vi "CRYAdd curve name.vi"(9 "Curent Name":u16(ring) caption="aa" items=["Recalled Curve1"], 10 "add/rename?":bool, 11 "Curve Names in":string[](array[string])) -> (3 "Curve Names out":string[](array[string]))   [LabVIEW 2013]
panel:
  out "dialog text":string
  in  "Cancel":bool
  in  "OK":bool
  in  "New":bool caption="aa"
  in  "Custom Name":string caption="aa"
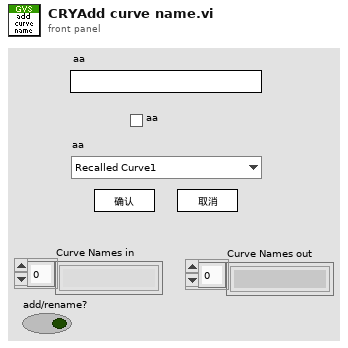
[diagram p1: front panel]
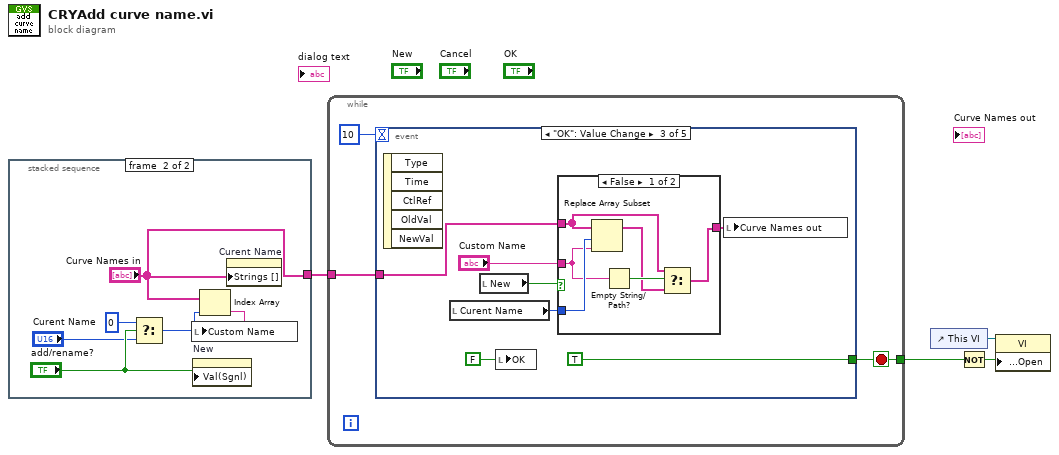
[diagram p0: block diagram]
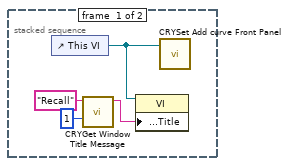
[diagram p2: hidden frame]
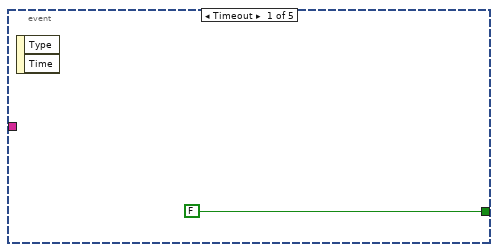
[diagram p3: hidden frame]
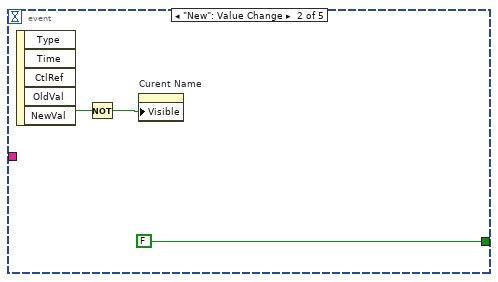
[diagram p4: hidden frame]
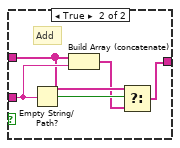
[diagram p5: hidden frame]
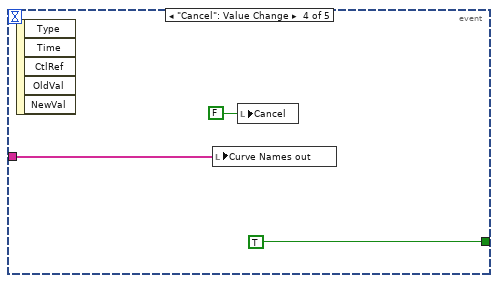
[diagram p6: hidden frame]
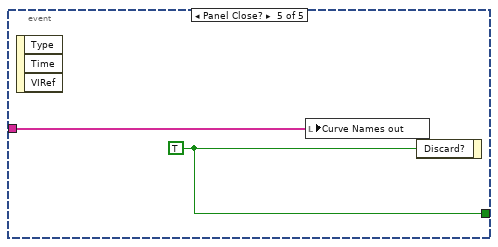
[diagram p7: hidden frame]
diagram:
  n1 = stacked-sequence {
    tunnel: [_ "Curve Names in"] -> w1
    frame #0 {
      n2 = control-ref of="This VI"() -> (w6:refnum<vi>)
      n3 = call "CRYGet Window Title Message.vi"("No"=1, "Kind"="Recall") -> ("Multibyte String"=w5:string)  [unwired: 4 in, 5 out]
      n4 = property class="VI"(reference=w6, "Front Panel.Title"=w5) -> ()  [unwired: 1 in, 2 out]
      n5 = call "CRYSet Add curve Front Panel.vi"("Vi Ref"=w6) -> ()  [unwired: 11 in]
    }
    frame #1 {
      n6 = Select(t=u16 0, s="add/rename?", f="Curent Name") -> (s? t:f=w9:u16)
      n7 = property on="New" class="Bool (strict)"("Val(Sgnl)"="add/rename?") -> ()  [unwired: 2 in, 2 out]
      n8 = Index Array(array="Curve Names in", index=w9) -> (element=w14:string)
      n9 = local write "Custom Name"(w14) -> ()
      n10 = property on="Curent Name" class="Ring (strict)"("Strings []"="Curve Names in") -> ()  [unwired: 2 in, 2 out]
    }
  }
  n11 = while {
    tunnel: [w16] -> w3
    tunnel: w1 -> [w15]
    stop <- w16 stop-if-true
    n12 = event shown="[2] \"OK\": Value Change" {
      selector: _ -> [_ _ _ _ _]
      dyn-events: _ -> [_ _ _ _ _]
      timeout: 10 -> [_ _ _ _ _]
      tunnel: [FALSE ("Discard?") FALSE ("Discard?") TRUE ("Discard?") TRUE ("Discard?") w44] -> w16
      tunnel: w15 -> [_ _ w22 w40 w43]
      event Timeout {
        n13 = event-data() -> ()  [unwired: 1 in, 2 out]
      }
      event "New": Value Change {
        n14 = event-data() -> ("NewVal"=w20:bool)  [unwired: 1 in, 4 out]
        n15 = Not(x=w20) -> (.not. x?=w21:bool)
        n16 = property on="Curent Name" class="Ring (strict)"("Visible"=w21) -> ()  [unwired: 2 in, 2 out]
      }
      event "OK": Value Change {
        n17 = event-data() -> ()  [unwired: 1 in, 5 out]
        n18 = local read "Curent Name"() -> (w25:u16)
        n19 = local read "New"() -> (w26:bool)
        n20 = local write "OK"(FALSE ("OK")) -> ()
        n21 = case shown="False" w26 {
          tunnel: w22 -> [w30 w37]
          tunnel: [w29 w35] -> w23
          tunnel: w25 -> [w34 _]
          tunnel: "Custom Name" -> [w33 w39]
          frame False {
            n22 = Replace Array Subset(array=w30, new element=w33, index=w34) -> (w31:string[])
            n23 = Empty String/Path?(string/path=w33) -> (empty?=w32:bool)
            n24 = Select(t=w30, s=w32, f=w31) -> (s? t:f=w29:string[])
          }
          frame True {
            # "Add"
            n25 = Empty String/Path?(string/path=w39) -> (empty?=w38:bool)
            n26 = Build Array (concatenate)(w37, w39) -> (w36:string[])
            n27 = Select(t=w37, s=w38, f=w36) -> (s? t:f=w35:string[])
          }
        }
        n28 = local write "Curve Names out"(w23) -> ()
      }
      event "Cancel": Value Change {
        n29 = event-data() -> ()  [unwired: 1 in, 5 out]
        n30 = local write "Curve Names out"(w40) -> ()
        n31 = local write "Cancel"(FALSE ("Cancel")) -> ()
      }
      event Panel Close? {
        w44 = TRUE ("Discard?")
        n32 = event-data() -> ()  [unwired: 1 in, 3 out]
        n33 = local write "Curve Names out"(w43) -> ()
        n34 = event-data("Discard?"=w44) -> ()  [unwired: 1 in, 1 out]
      }
    }
  }
  n35 = control-ref of="This VI"() -> (w4:refnum<vi>)
  n36 = Not(x=w3) -> (.not. x?=w2:bool)
  n37 = property class="VI"(reference=w4, "Front Panel.Open"=w2) -> ()  [unwired: 1 in, 2 out]
